vi "GetSelItemTag.vi"(8 "error in (no error)":errorcluster, 11 "CMenu in":refnum<class "CMenu.lvclass">) -> (0 "error out":errorcluster, 2 "SelItemTag":string, 3 "CMenu out":refnum<class "CMenu.lvclass">)   [LabVIEW 2020, in "CMenu.lvclass"]
uses:
  CMenu.lvclass
  CMenu.lvclass/CMenu.ctl
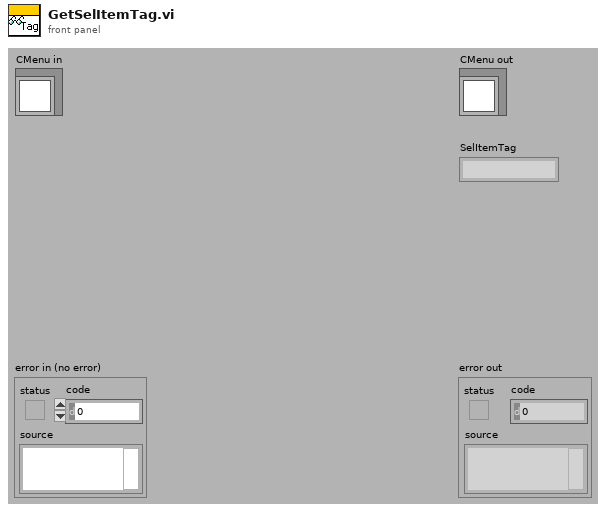
[diagram p1: front panel]
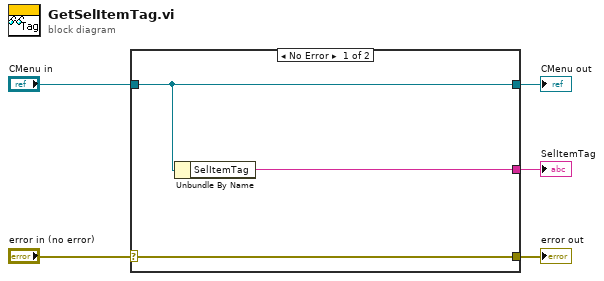
[diagram p0: block diagram]
diagram:
  n1 = case shown="No Error" "error in (no error)" {
    selector: "error in (no error)" -> [w8 w9]
    tunnel: [w8 w9] -> w4
    tunnel: [w7 w10] -> w2
    tunnel: "CMenu in" -> [w7 w10]
    tunnel: [w6 _] -> w1
    frame No Error {
      n2 = Unbundle By Name(w7) -> ("SelItemTag"=w6:string)
    }
    frame Error {
    }
  }
  "error out" <- w4
  "CMenu out" <- w2
  "SelItemTag" <- w1
